vi "Drive Backward V.3.0.vi"(8 "Desired Angle":dbl, 11 "Encoder Distance (in.)":dbl) -> (3 "Stop":bool)   [LabVIEW 2017]
uses:
  Robot Global Data V.3.0.vi
panel:
  out "Gyro":cluster{"Gyro":dbl, dbl}(graph)
  out "Drive Speeds":cluster{dbl, dbl}(graph)
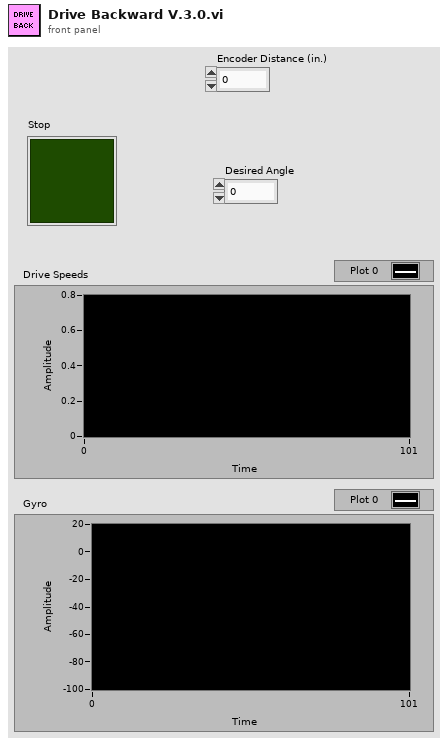
[diagram p1: front panel]
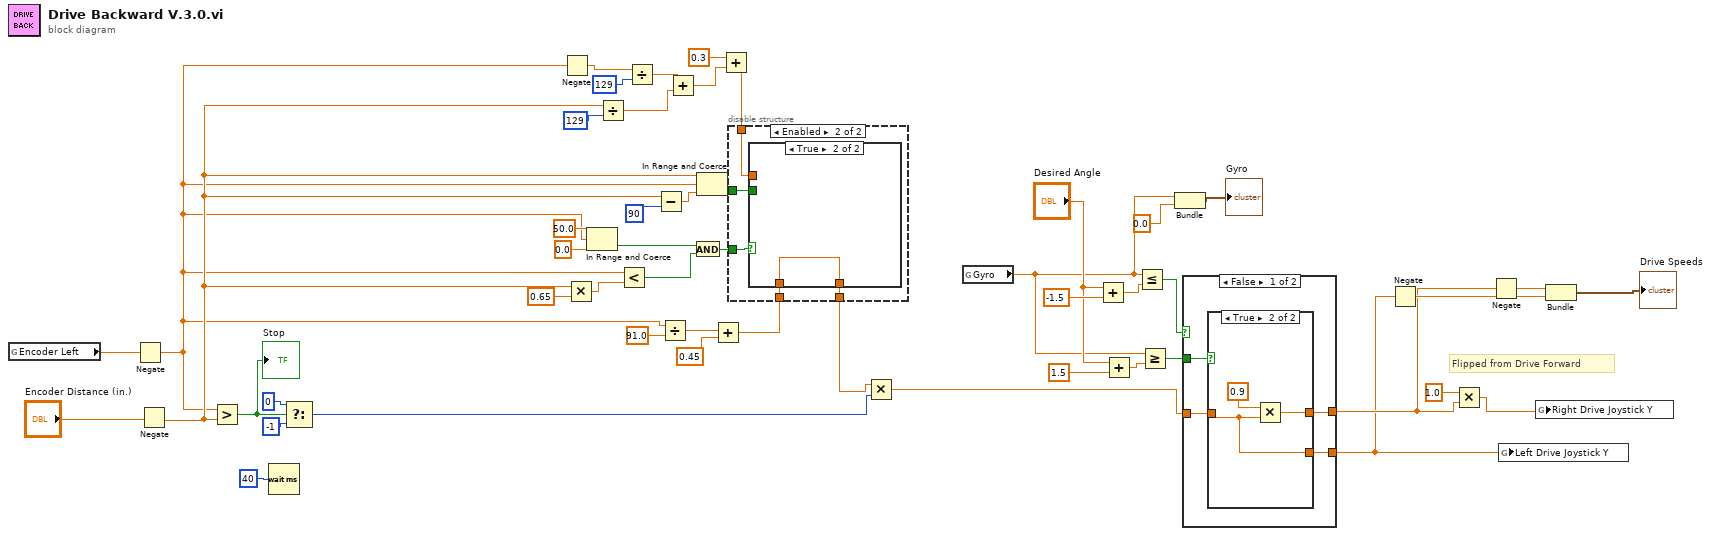
[diagram p0: block diagram]
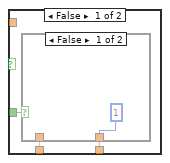
[diagram p3: hidden frame]
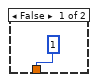
[diagram p6: hidden frame]
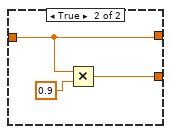
[diagram p8: hidden frame]
diagram:
  # "Flipped from Drive Forward"
  n1 = global read "Robot Global Data V.3.0.vi" "Encoder Left"() -> (w25:dbl)
  n2 = Negate(x=w25) -> (-x=w2:dbl)
  n3 = Negate(x="Encoder Distance (in.)") -> (-x=w5:dbl)
  n4 = Greater?(x=w2, y=w5) -> (0:w48:bool)
  "Stop" <- w48
  n5 = Wait (ms)(milliseconds to wait=u32 40) -> ()  [unwired: 1 out]
  n6 = Select(t=0, s=w48, f=-1) -> (s? t:f=w27:i32)
  n7 = Negate(x=w2) -> (-x=w44:dbl)
  n8 = Multiply(x=w5, y=0.65) -> (x*y=w3:dbl)
  n9 = In Range and Coerce(upper limit=50.0, x=w2, lower limit=0.0) -> (In Range?=w7:bool)  [unwired: 1 out]
  n10 = Divide(x=w5, y=129) -> (x/y=w42:dbl)
  n11 = Less?(x=w2, y=w3) -> (x < y?=w1:bool)
  n12 = Divide(x=w44, y=129) -> (x/y=w41:dbl)
  n13 = Subtract(x=w5, y=90) -> (x-y=w39:dbl)
  n14 = Divide(x=w2, y=91.0) -> (x/y=w34:dbl)
  n15 = Add(x=w41, y=w42) -> (x+y=w31:dbl)
  n16 = And(x=w7, y=w1) -> (x .and. y?=w8:bool)
  n17 = In Range and Coerce(upper limit=w5, x=w2, lower limit=w39) -> (In Range?=w38:bool)  [unwired: 1 out]
  n18 = Add(x=w34, y=0.45) -> (x+y=w32:dbl)
  n19 = Add(x=0.3, y=w31) -> (x+y=w29:dbl)
  n20 = disable-structure shown="Enabled" {
    disable-tunnel: w38 -> [w55 w65]
    disable-tunnel: w8 -> [w54 w62]
    disable-tunnel: w32 -> [w53 w66]
    disable-tunnel: w29 -> [w52 w64]
    disable-tunnel: [w51 w63] -> w28
    frame Disabled {
      n21 = case shown="True" w55 {
        tunnel: w52 -> [_ w61]
        tunnel: [w57 w61] -> w51
        tunnel: w54 -> [w58 _]
        tunnel: w53 -> [w56 _]
        frame False {
          n22 = case shown="False" w58 {
            tunnel: [1 w60] -> w57
            tunnel: w56 -> [_ w60]
            frame False {
            }
            frame True {
            }
          }
        }
        frame True {
        }
      }
    }
    frame Enabled {
      n23 = case shown="True" w62 {
        tunnel: [w70 w73] -> w63
        tunnel: w66 -> [w69 w73]
        tunnel: w65 -> [w68 _]
        tunnel: w64 -> [w67 _]
        frame False {
          n24 = case shown="True" w68 {
            tunnel: [1 w72] -> w70
            tunnel: w69 -> [_ _]
            tunnel: w67 -> [_ w72]
            frame False {
            }
            frame True {
            }
          }
        }
        frame True {
        }
      }
    }
  }
  n25 = Multiply(x=w28, y=w27) -> (x*y=w26:dbl)
  n26 = global read "Robot Global Data V.3.0.vi" "Gyro"() -> (w14:dbl)
  n27 = Add(x="Desired Angle", y=-1.5) -> (x+y=w22:dbl)
  n28 = Add(x="Desired Angle", y=1.5) -> (x+y=w21:dbl)
  n29 = Less Or Equal?(x=w14, y=w22) -> (x <= y?=w46:bool)
  n30 = Greater Or Equal?(x=w14, y=w21) -> (x >= y?=w45:bool)
  n31 = Bundle("Gyro"=w14, 0.0) -> (→"Gyro":cluster{"Gyro":dbl, dbl})  [unwired: 1 in]
  n32 = case shown="False" w46 {
    tunnel: [w74 w83] -> w12
    tunnel: [w75 w82] -> w9
    tunnel: w26 -> [w76 w83]
    tunnel: w45 -> [w77 _]
    frame False {
      n33 = case shown="True" w77 {
        tunnel: w76 -> [w78 w80]
        tunnel: [w78 w80] -> w75
        tunnel: [w78 w79] -> w74
        frame False {
        }
        frame True {
          n34 = Multiply(x=0.9, y=w80) -> (x*y=w79:dbl)
        }
      }
    }
    frame True {
      n35 = Multiply(x=w83, y=0.9) -> (x*y=w82:dbl)
    }
  }
  n36 = Negate(x=w9) -> (-x=w16:dbl)
  n37 = Multiply(x=1.0, y=w12) -> (x*y=w10:dbl)
  n38 = Negate(x=w12) -> (-x=w17:dbl)
  n39 = global write "Robot Global Data V.3.0.vi" "Left Drive Joystick Y"(w9) -> ()
  n40 = global write "Robot Global Data V.3.0.vi" "Right Drive Joystick Y"(w10) -> ()
  n41 = Bundle(w17, w16) -> (→"Drive Speeds":cluster{dbl, dbl})  [unwired: 1 in]
